vi "Grover search.vi"   [LabVIEW 2016]
uses:
  Gates/Polymorph/Xsingle.vi
  Gates/Polymorph/Xtarget.vi
  Probes/Polymorph/P bar graph.vi
panel:
  # "4-qubit Grover Search Example"
  # "*Open the block diagram for the circuit view (Ctrl+E)"
types:
  T1 = typedef "Circuit Cluster.ctl" = cluster{"Loop No":i32, "Wire":cluster{"No":i32, "Depth":i32, "Hold":i32[][], "Permits":refnum<notifier>}, "Size":refnum<queue>, "Composition":refnum<queue>, "Gate class":refnum<class "GateAbst.lvclass">}
  T2 = typedef "Controls.ctl" = i32[][]
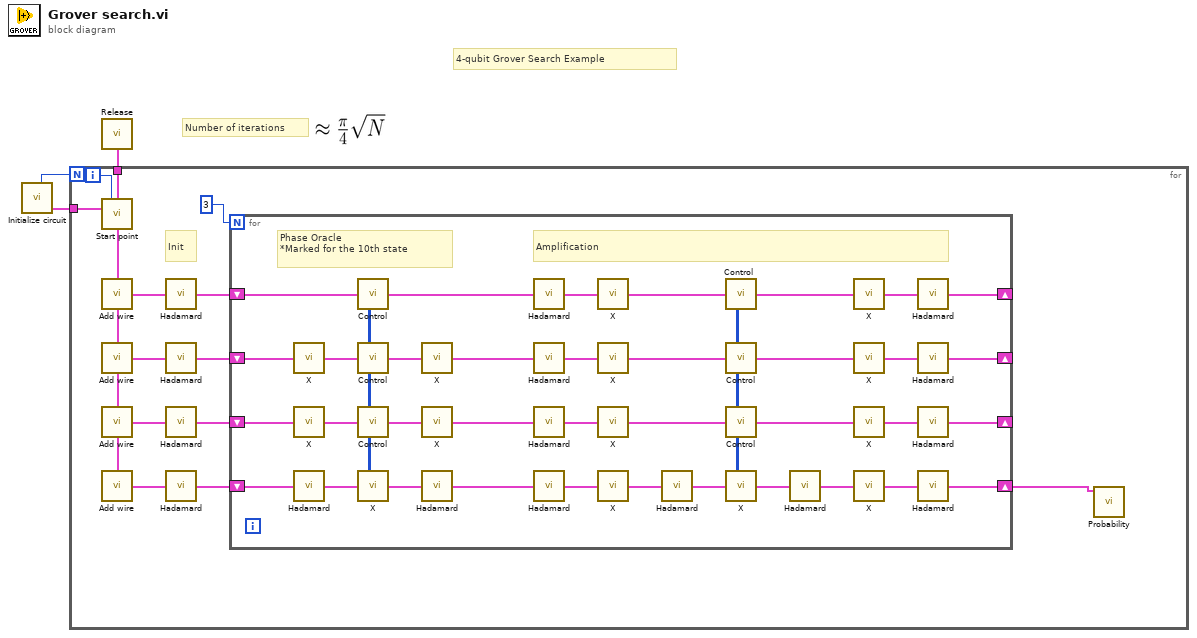
[diagram p0: block diagram]
diagram:
  # "4-qubit Grover Search Example"
  # "Number of iterations"
  n1 = call "Initialize circuit.vi"() -> ("N"=w2:i32, "Circuit cluster"=w3:T1)  [unwired: 8 in]
  n2 = for {
    N: w2 -> [_]
    tunnel: w3 -> [w11]
    tunnel: [w5] -> w1
    i -> [w4]
    # "Init"
    n3 = call "Start point.vi"("Loop No"=w4, "Circuit cluster in"=w11) -> ("Up circuit cluster out"=w5:T1, "Down circuit cluster out"=w9:T1)  [unwired: 12 in]
    n4 = call "Add wire.vi"("Circuit cluster in"=w9) -> ("Wire out"=w16:T1, "Circuit cluster out"=w20:T1)  [unwired: 13 in]
    n5 = call "Add wire.vi"("Circuit cluster in"=w20) -> ("Wire out"=w17:T1, "Circuit cluster out"=w19:T1)  [unwired: 13 in]
    n6 = call "Add wire.vi"("Circuit cluster in"=w19) -> ("Wire out"=w18:T1, "Circuit cluster out"=w10:T1)  [unwired: 13 in]
    n7 = call "Add wire.vi"("Circuit cluster in"=w10) -> ("Wire out"=w8:T1)  [unwired: 13 in, 1 out]
    n8 = call "Hadamard.vi"("Wire in"=w16) -> ("Wire out"=w14:T1)  [unwired: 4 in]
    n9 = call "Hadamard.vi"("Wire in"=w17) -> ("Wire out"=w13:T1)  [unwired: 4 in]
    n10 = call "Hadamard.vi"("Wire in"=w18) -> ("Wire out"=w15:T1)  [unwired: 4 in]
    n11 = call "Hadamard.vi"("Wire in"=w8) -> ("Wire out"=w7:T1)  [unwired: 4 in]
    n12 = for {
      N: 3 -> [_]
      shift-right: [w62] -> _
      shift-left: w15 -> [w60]
      shift-right: [w37] -> _
      shift-left: w14 -> [w61]
      shift-right: [w36] -> _
      shift-left: w13 -> [w32]
      shift-right: [w33] -> w6
      shift-left: w7 -> [w58]
      # "Amplification"
      # "Phase Oracle\n*Marked for the 10th state"
      n13 = call-poly "X.vi"("Wire in"=w32) -> ("Wire out"=w31:T1)  [unwired: 8 in]
      n14 = call-poly "X.vi"("Wire in"=w60) -> ("Wire out"=w59:T1)  [unwired: 8 in]
      n15 = call "Hadamard.vi"("Wire in"=w58) -> ("Wire out"=w57:T1)  [unwired: 4 in]
      n16 = call "Control.vi"("Wire in"=w61) -> ("uc OUT"=w26:T2, "Wire out"=w27:T1)  [unwired: 6 in, 1 out]
      n17 = call "Control.vi"("uc IN"=w26, "Wire in"=w31) -> ("uc OUT"=w25:T2, "Wire out"=w30:T1)  [unwired: 5 in, 1 out]
      n18 = call "Control.vi"("uc IN"=w25, "Wire in"=w59) -> ("uc OUT"=w24:T2, "Wire out"=w55:T1)  [unwired: 5 in, 1 out]
      n19 = call-poly "X.vi"("Up control in"=w24, "Wire in"=w57) -> ("Wire out"=w56:T1)  [unwired: 7 in]
      n20 = call-poly "X.vi"("Wire in"=w30) -> ("Wire out"=w29:T1)  [unwired: 8 in]
      n21 = call-poly "X.vi"("Wire in"=w55) -> ("Wire out"=w35:T1)  [unwired: 8 in]
      n22 = call "Hadamard.vi"("Wire in"=w56) -> ("Wire out"=w34:T1)  [unwired: 4 in]
      n23 = call "Hadamard.vi"("Wire in"=w27) -> ("Wire out"=w52:T1)  [unwired: 4 in]
      n24 = call "Hadamard.vi"("Wire in"=w29) -> ("Wire out"=w49:T1)  [unwired: 4 in]
      n25 = call "Hadamard.vi"("Wire in"=w35) -> ("Wire out"=w48:T1)  [unwired: 4 in]
      n26 = call "Hadamard.vi"("Wire in"=w34) -> ("Wire out"=w47:T1)  [unwired: 4 in]
      n27 = call-poly "X.vi"("Wire in"=w52) -> ("Wire out"=w51:T1)  [unwired: 8 in]
      n28 = call-poly "X.vi"("Wire in"=w49) -> ("Wire out"=w28:T1)  [unwired: 8 in]
      n29 = call-poly "X.vi"("Wire in"=w48) -> ("Wire out"=w50:T1)  [unwired: 8 in]
      n30 = call-poly "X.vi"("Wire in"=w47) -> ("Wire out"=w46:T1)  [unwired: 8 in]
      n31 = call "Hadamard.vi"("Wire in"=w46) -> ("Wire out"=w45:T1)  [unwired: 4 in]
      n32 = call "Control.vi"("Wire in"=w51) -> ("uc OUT"=w23:T2, "Wire out"=w39:T1)  [unwired: 6 in, 1 out]
      n33 = call "Control.vi"("uc IN"=w23, "Wire in"=w28) -> ("uc OUT"=w22:T2, "Wire out"=w40:T1)  [unwired: 5 in, 1 out]
      n34 = call "Control.vi"("uc IN"=w22, "Wire in"=w50) -> ("uc OUT"=w21:T2, "Wire out"=w44:T1)  [unwired: 5 in, 1 out]
      n35 = call-poly "X.vi"("Up control in"=w21, "Wire in"=w45) -> ("Wire out"=w54:T1)  [unwired: 7 in]
      n36 = call "Hadamard.vi"("Wire in"=w54) -> ("Wire out"=w53:T1)  [unwired: 4 in]
      n37 = call-poly "X.vi"("Wire in"=w39) -> ("Wire out"=w38:T1)  [unwired: 8 in]
      n38 = call-poly "X.vi"("Wire in"=w40) -> ("Wire out"=w41:T1)  [unwired: 8 in]
      n39 = call-poly "X.vi"("Wire in"=w44) -> ("Wire out"=w43:T1)  [unwired: 8 in]
      n40 = call-poly "X.vi"("Wire in"=w53) -> ("Wire out"=w42:T1)  [unwired: 8 in]
      n41 = call "Hadamard.vi"("Wire in"=w38) -> ("Wire out"=w37:T1)  [unwired: 4 in]
      n42 = call "Hadamard.vi"("Wire in"=w41) -> ("Wire out"=w36:T1)  [unwired: 4 in]
      n43 = call "Hadamard.vi"("Wire in"=w43) -> ("Wire out"=w62:T1)  [unwired: 4 in]
      n44 = call "Hadamard.vi"("Wire in"=w42) -> ("Wire out"=w33:T1)  [unwired: 4 in]
    }
    n45 = call-poly "Probability.vi"("Wire in"=w6) -> ()  [unwired: 11 in]
  }
  n46 = call "Release.vi"("Circuit cluster in"=w1) -> ()  [unwired: 15 in]
